vi "Init.vi"(8 "error in (no error)":errorcluster) -> (0 "error out":errorcluster, 3 "VideoMux out":refnum<class "VideoMux.lvclass">)   [LabVIEW 2022 SP3, in "VideoMux.lvlib" / "VideoMux.lvclass"]
uses:
  VideoMux.lvclass
  VideoMux.lvclass/VideoMux.ctl
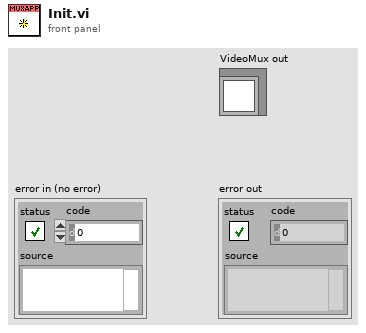
[diagram p1: front panel]
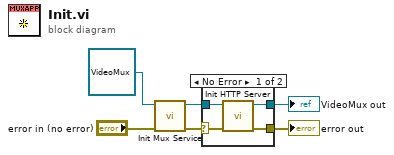
[diagram p0: block diagram]
diagram:
  n1 = call "Init Mux Service.vi"("error in (no error)"="error in (no error)", "VideoMux in"=refnum<class "VideoMux.lvclass"> refnum) -> ("error out"=w5:errorcluster, "VideoMux out"=w2:refnum<class "VideoMux.lvclass">)  [unwired: 8 in]
  n2 = case shown="No Error" w5 {
    selector: w5 -> [w10 w11]
    tunnel: [w9 w11] -> w3
    tunnel: w2 -> [w8 w12]
    tunnel: [w7 w12] -> w1
    frame No Error {
      n3 = call "Init HTTP Server.vi"("error in (no error)"=w10, "VideoMux in"=w8) -> ("error out"=w9:errorcluster, "VideoMux out"=w7:refnum<class "VideoMux.lvclass">)  [unwired: 8 in]
    }
    frame Error {
    }
  }
  "error out" <- w3
  "VideoMux out" <- w1
